vi "ActorPlugin-003-CreateWorkOrder.vi"(0 "FTW Actor Instance Configuration":string="{\n  \"Identity\": \"ActorName\",\n  \"InboxAddress\": \"tcp://127.0.0.1:*\",\n  \"PublisherAddress\": \"tcp://127.0.0.1:*\",\n  \"DebugEnableInboxLogging\": false,\n  \"DebugEnableJobLogging\": false,\n  \"DebugShowPanel\": false\n}", 11 "error in":errorcluster) -> (15 "Error":errorcluster)   [LabVIEW 2013, in "ERP-CreateWorkOrder.lvclass"]
uses:
  Actors/ERP-Create Work Order/ERP-CreateWorkOrder.lvclass
  Actors/ERP-Create Work Order/Controls/Cntrl-LoadPartNumbers.ctl
  Actors/ERP-Create Work Order/Controls/Cntrl-CreateWorkOrder.ctl
  Actors/ERP-Create Work Order/Controls/Cntrl-ClearWorkOrderVariables.ctl
  Actors/ERP-Create Work Order/ERP-CreateWorkOrder.lvclass/ERP-CreateWorkOrder.ctl
  <userlib>/_OpenG.lib/array/array.llb/Reorder 2D Array2 (String)__ogtk.vi
  ftw-dataflow/Actor/src/Instance/FTW-ActorInstance.lvclass
  ftw-dataflow/Actor/src/Message/Request/FTW-Message-IncomingRequest.lvclass
  ERP-ConfigPageNewFeather/PCert-ConfigPageNF.lvclass
panel:
  in  "Choose Part Number*":u16(ring)
  in  "Clear Work Order Variables":T1
  in  "Load Part Numbers":T2
  in  "Attach Special Instructions (Word or PDF files only!!) 2":path
  in  "Due Date*":timestamp format="%<%x>T"
  in  "Start Date*":timestamp format="%<%x>T"
  in  "Attach Special Instructions (Word or PDF files only!!) 1":path
  in  "Note - Special Instructions":string
  in  "Stage Deployment for Part":u16(ring) items=["Standard Part", "Non-Standard Part", "Inventory Part", "Waiting for Customer Supplied Material", "RMA"]
  in  "Unique Identifier":u16(ring) items=["", "Cascade", "Feinmetall", "Hermes", "Jem", "T.I.P.S"]
  in  "Type Part Number*":string
  out "Part Number Description":string
  in  "Quantity to Make*":i32
  in  "Customer*":string
  in  "Validate Typed Number":bool
  in  "Sales Order*":string
  in  "Create Work Order":T3
  # "Please Fill Out the Below Information to Create a work Order"
  # "*=Required"
  # "1."
  # "2."
  # "3."
  # "5."
  # "4."
  # "Under Construction Currently\nDoes not Work!"
  # "6."
  # "7."
  # "Drag and Drop or Select the Files to Attach"
  # "8."
  # "9."
  # "Inputs"
  # "Outputs"
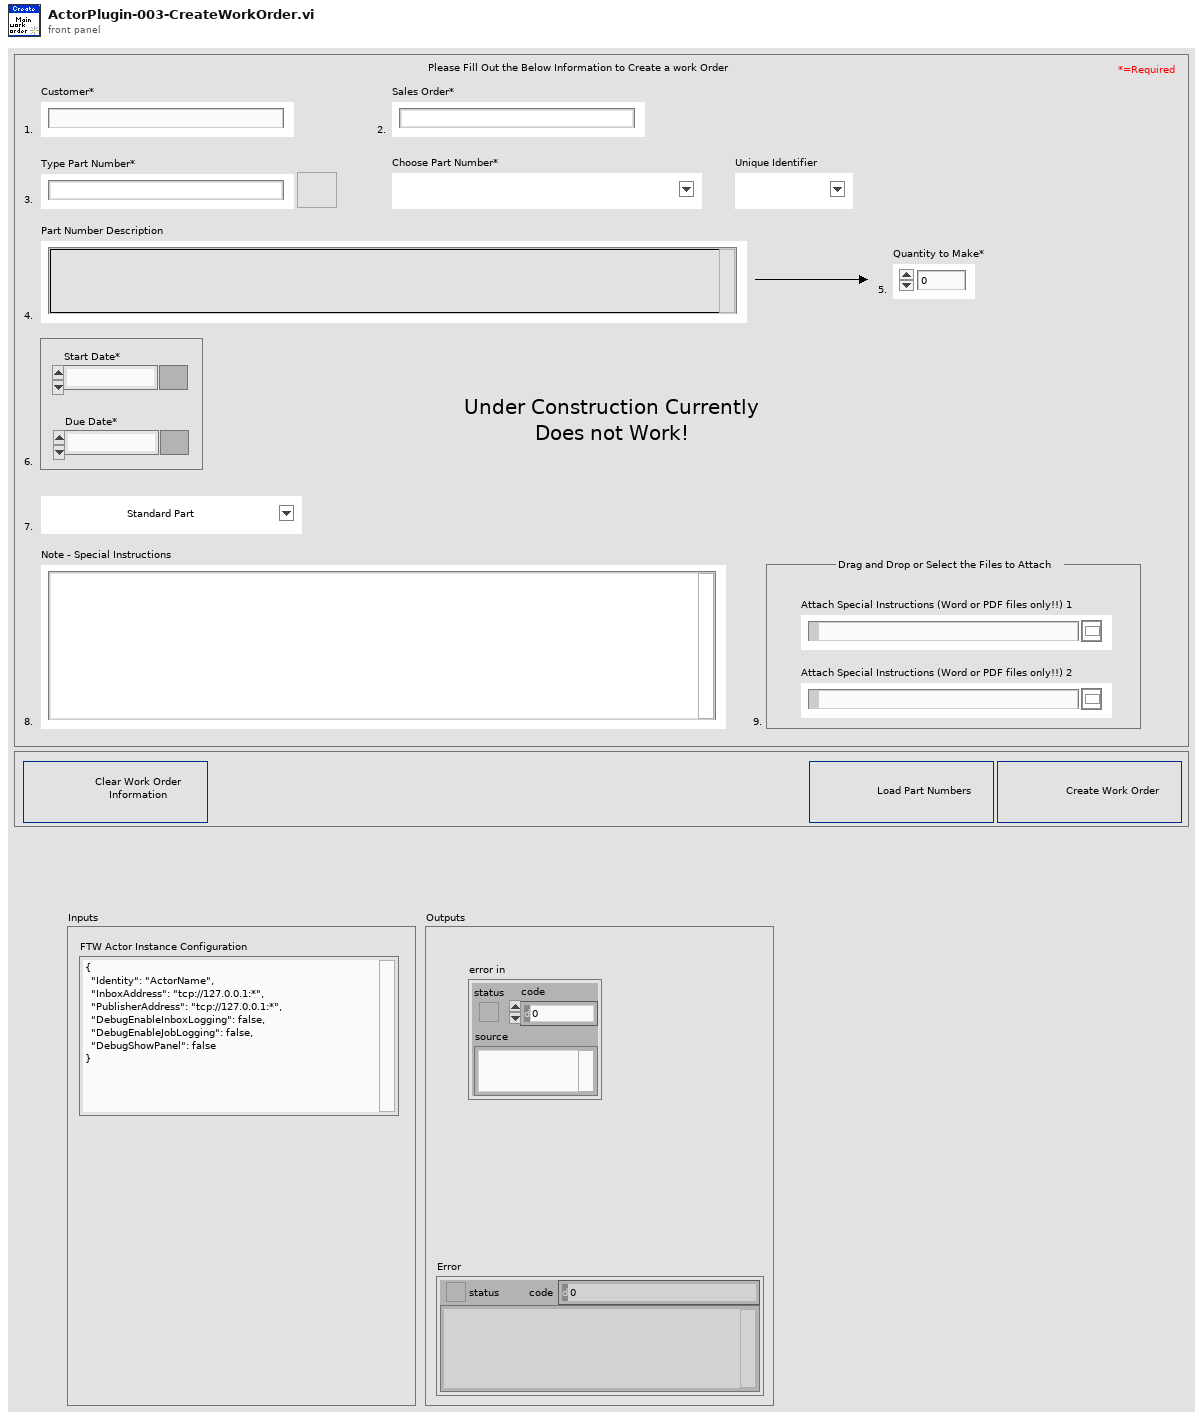
[diagram p1: front panel]
types:
  T1 = typedef "Cntrl-ClearWorkOrderVariables.ctl" = bool
  T2 = typedef "Cntrl-LoadPartNumbers.ctl" = bool
  T3 = typedef "Cntrl-CreateWorkOrder.ctl" = bool
  T4 = cluster{"Incoming Requests":refnum<event-registration>, "Additional Registration Types":refnum<event-registration>}
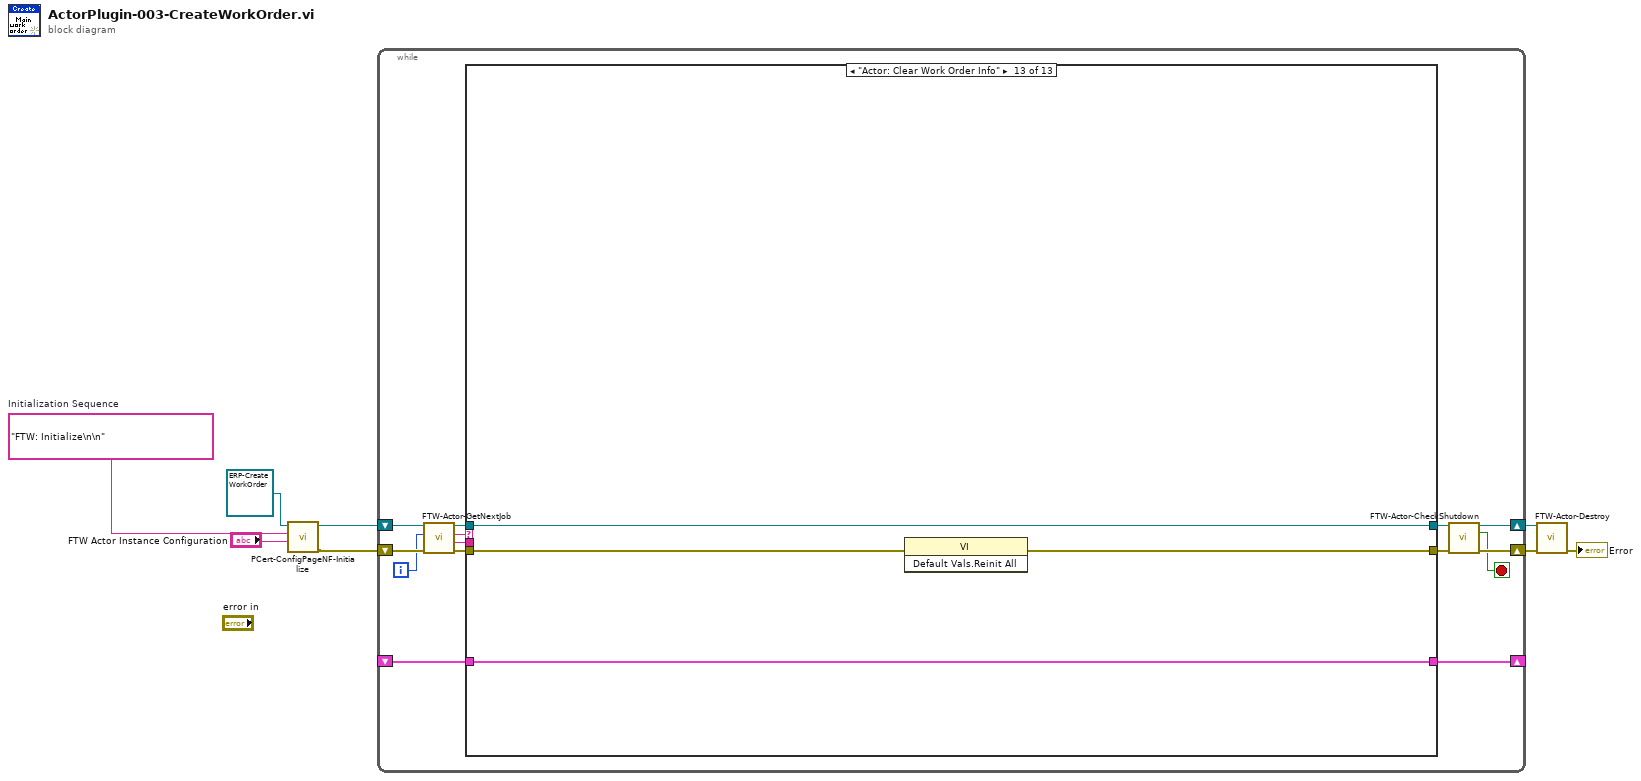
[diagram p0: block diagram]
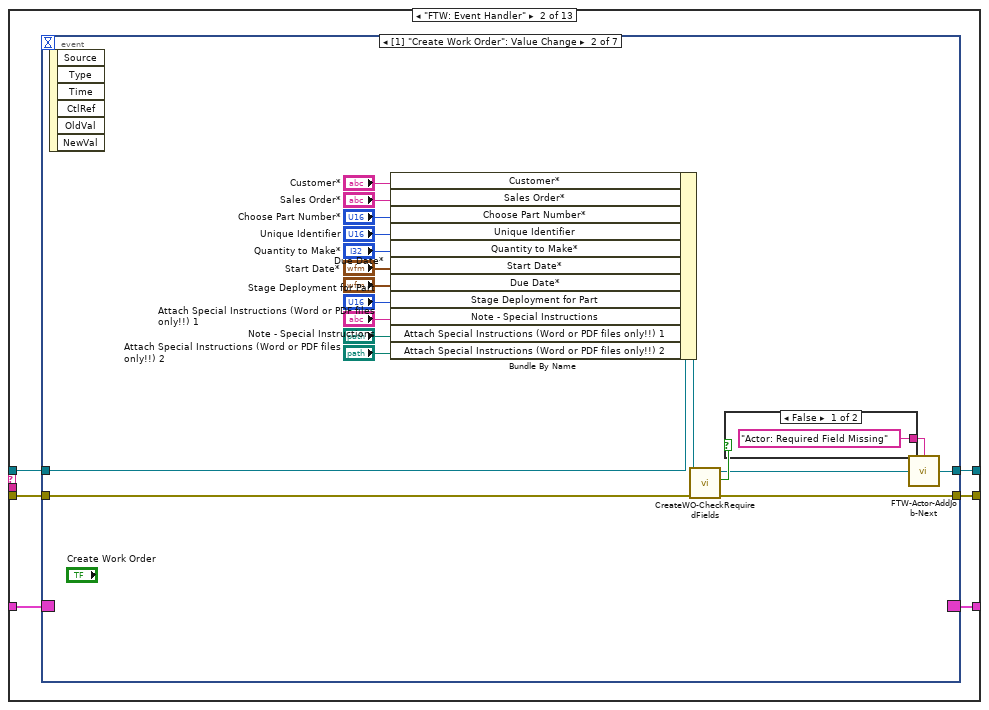
[diagram p3: hidden frame]
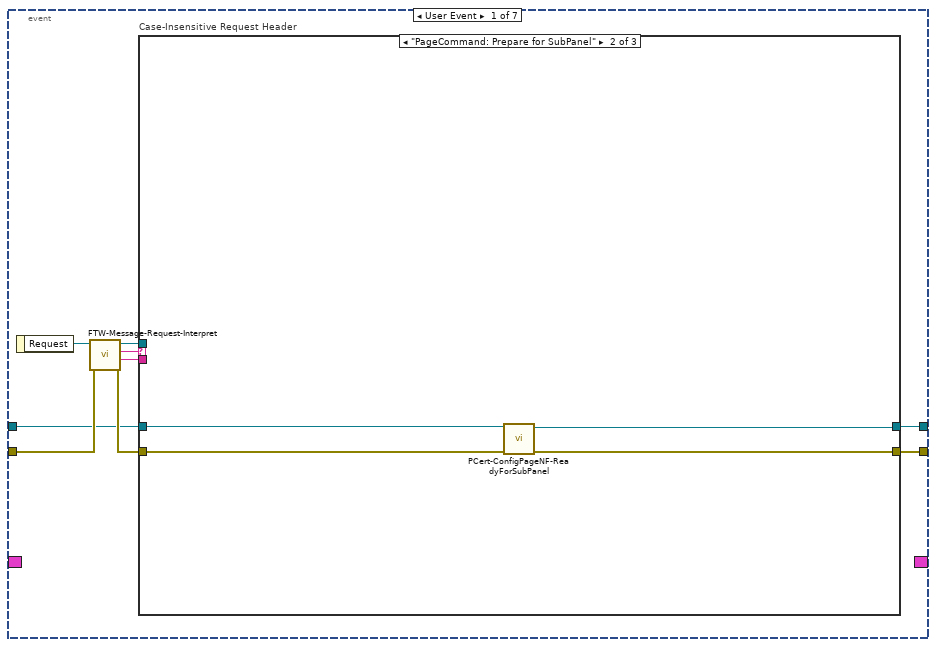
[diagram p4: hidden frame]
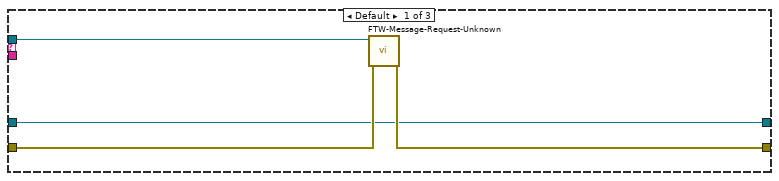
[diagram p5: hidden frame]
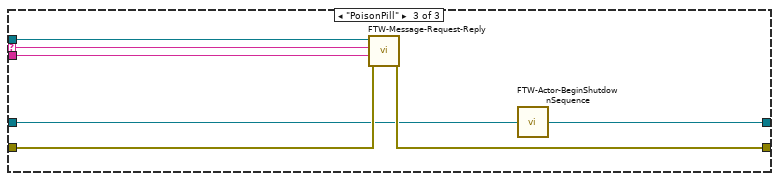
[diagram p6: hidden frame]
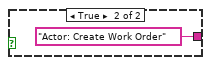
[diagram p7: hidden frame]
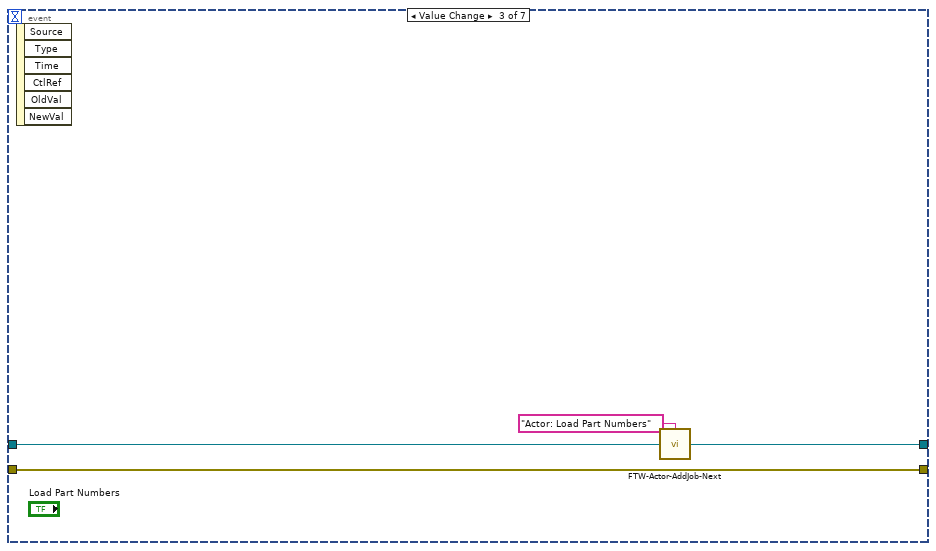
[diagram p8: hidden frame]
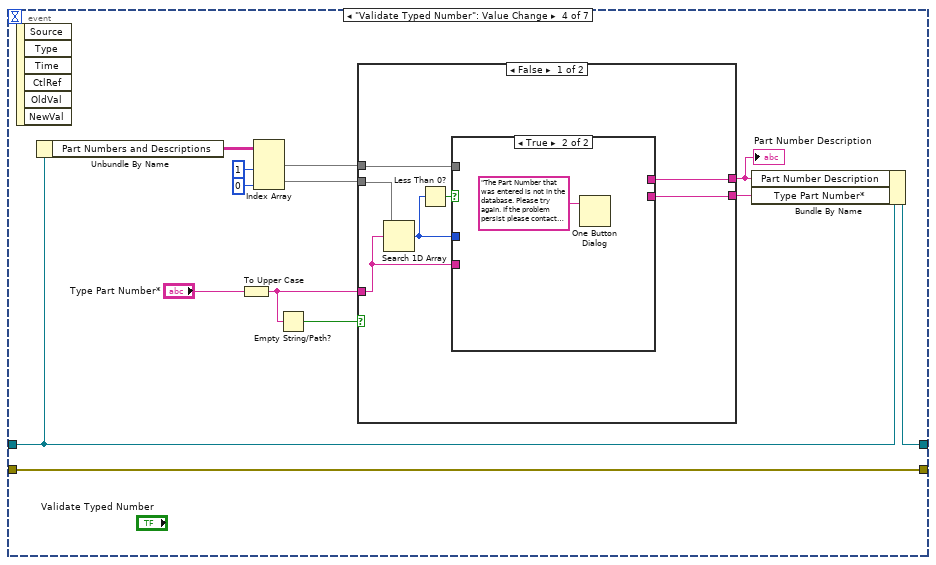
[diagram p9: hidden frame]
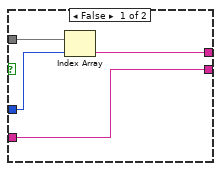
[diagram p10: hidden frame]
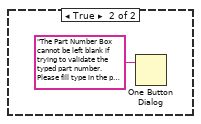
[diagram p11: hidden frame]
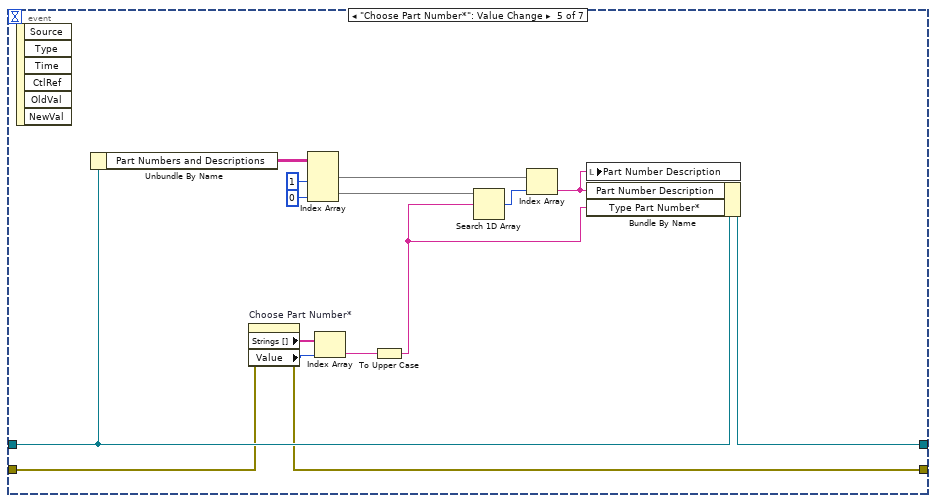
[diagram p12: hidden frame]
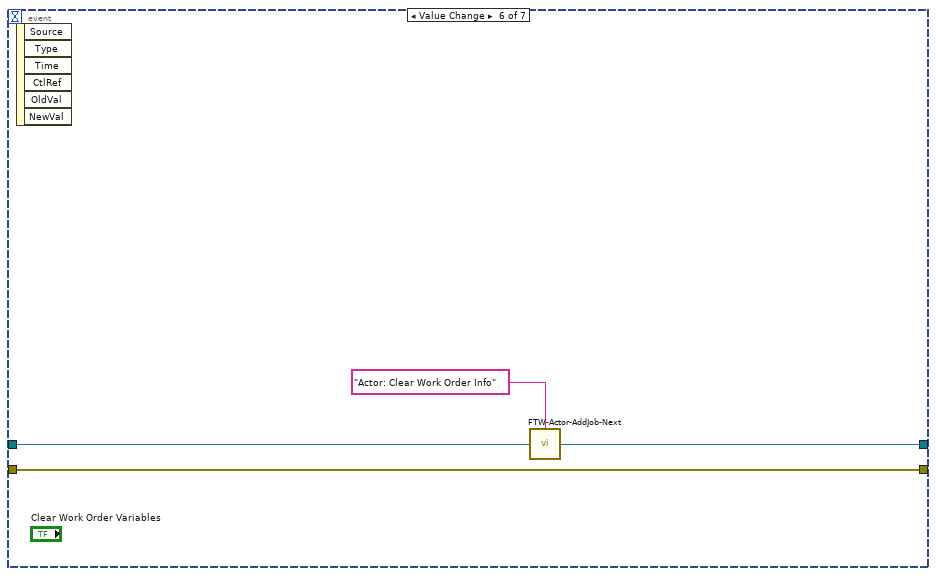
[diagram p13: hidden frame]
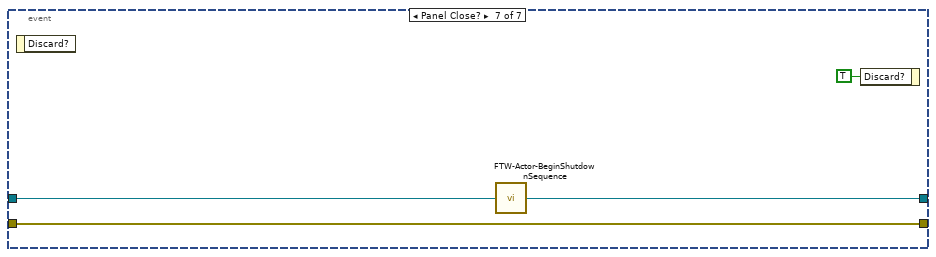
[diagram p14: hidden frame]
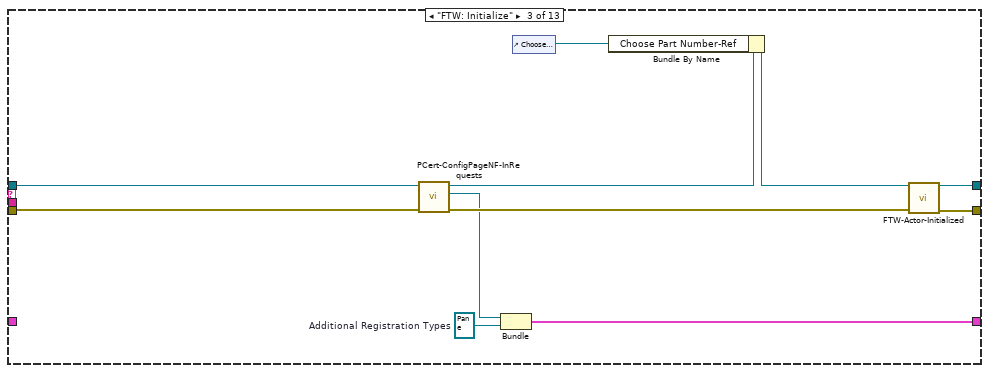
[diagram p15: hidden frame]
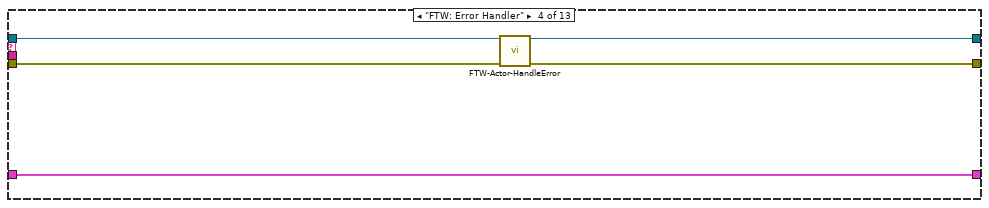
[diagram p16: hidden frame]
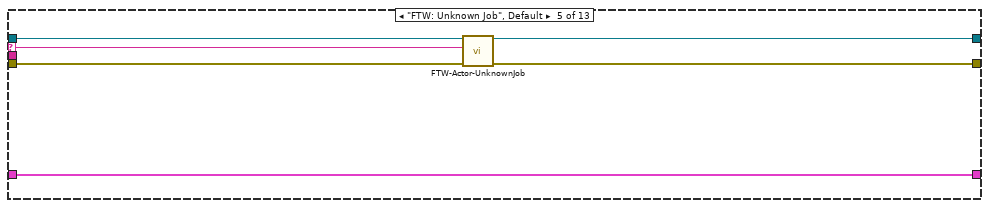
[diagram p17: hidden frame]
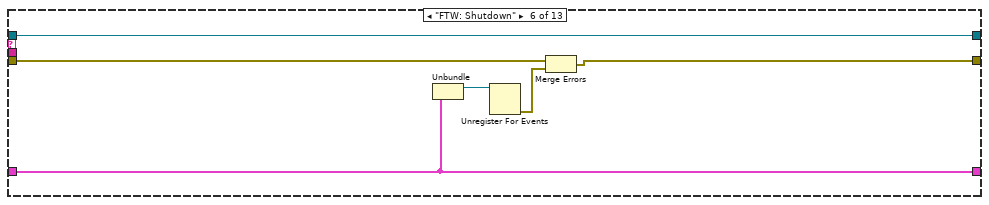
[diagram p18: hidden frame]
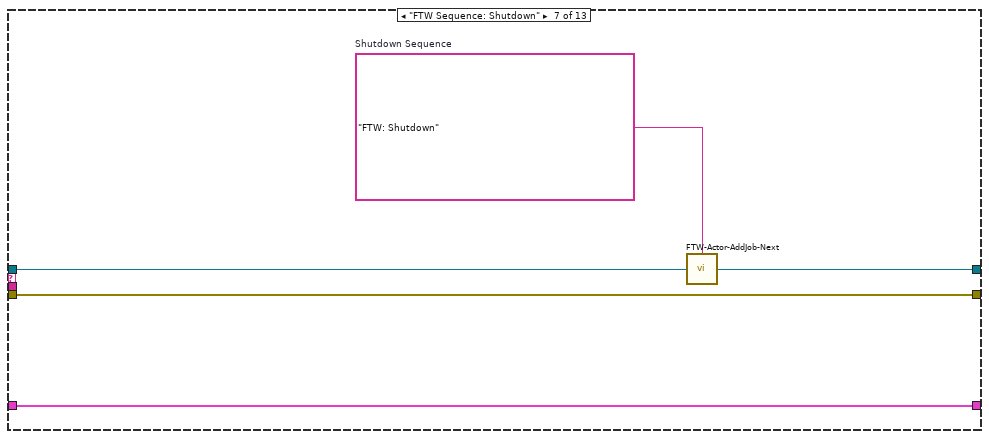
[diagram p19: hidden frame]
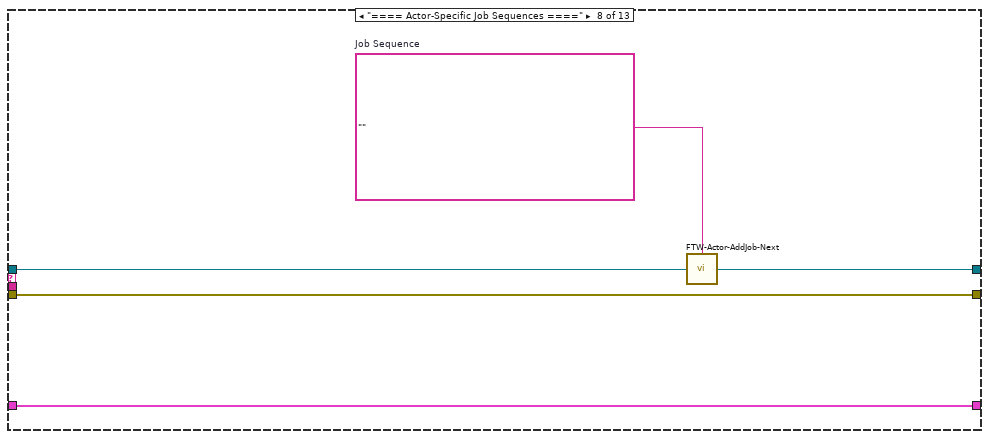
[diagram p20: hidden frame]
diagram:
  w5 = "FTW: Initialize\n\n"  # Initialization Sequence
  n1 = call-dynamic "PCert-ConfigPageNF-Initialize.vi"("FTW Actor Instance Configuration"="FTW Actor Instance Configuration", "Initialization Job Sequence"=w5, "ERP-ConfigPageNF.lvclass"=refnum<class "ERP-CreateWorkOrder.lvclass"> refnum ("ERP-CreateWorkOrder.lvclass")) -> ("error out"=w3:errorcluster, "ERP-ConfigPageNF out"=w4:refnum<class "ERP-CreateWorkOrder.lvclass">)  [unwired: 7 in]
  n2 = while {
    shift-right: [w12] -> w7
    shift-left: w3 -> [w19]
    shift-right: [w9] -> _
    shift-left: _ -> [w22]
    shift-right: [w14] -> w8
    shift-left: w4 -> [w21]
    i -> [w10]
    stop <- w11 stop-if-true
    n3 = call "FTW-Actor-GetNextJob.vi"("error in"=w19, "Jobs Performed"=w10, "FTW Actor Instance"=w21) -> ("error out"=w18:errorcluster, "Job Data"=w16:string, "Job Name"=w17:string, "FTW Actor Instance out"=w20:refnum<class "ERP-CreateWorkOrder.lvclass">)  [unwired: 5 in]
    n4 = case shown="\"Actor: Clear Work Order Info\"" w17 {
      selector: w17 -> [_ _ _ _ w146 _ _ _ _ _ _ _ _]
      tunnel: [w24 w31 w139 w141 w149 w155 w161 w166 w170 w175 w221 w224 w259] -> w13
      tunnel: w18 -> [w24 w30 w137 w143 w150 w152 w161 w166 w170 w178 w222 w233 w260]
      tunnel: w22 -> [w25 w26 _ w145 w151 w157 w162 w167 w169 w186 w223 w235 w262]
      tunnel: [w25 w29 w133 w145 w151 w157 w162 w167 w169 w186 w223 w235 w262] -> w9
      tunnel: w16 -> [_ _ _ _ _ _ _ _ _ _ _ _ _]
      tunnel: [w23 w28 w140 w142 w147 w153 w159 w164 w168 w174 w219 w225 w261] -> w15
      tunnel: w20 -> [w23 w27 w138 w144 w148 w153 w160 w165 w168 w179 w220 w234 w261]
      frame "==== Featherweight Framework Jobs ====" {
      }
      frame "FTW: Event Handler" {
        n5 = event shown="[1] \"Create Work Order\": Value Change" {
          selector: w26 -> [_ _ _ _ _ _ _]
          dyn-events: [_ _ _ _ _ _ _] -> w29
          timeout: _ -> [_ _ _ _ _ _ _]
          tunnel: [w37 w71 w80 w81 w107 w125 w128] -> w31
          tunnel: w30 -> [w38 w72 w80 w81 w109 w125 w128]
          tunnel: [w36 w58 w77 w87 w112 w122 w126] -> w28
          tunnel: w27 -> [w35 w74 w78 w88 w113 w123 w127]
          event User Event {
            n6 = event-data() -> ("Request"=w39:refnum<class "FTW-Message-IncomingRequest.lvclass">)  [unwired: 1 in]
            n7 = call "FTW-Message-Request-Interpret.vi"("error in"=w38, "FTW Incoming Request"=w39) -> ("error out"=w40:errorcluster, "Request Body"=w33:string, "Request Header"=w34:string, "FTW Incoming Request out"=w32:refnum<class "FTW-Message-IncomingRequest.lvclass">)  [unwired: 6 in]
            n8 = case "Case-Insensitive Request Header" shown="\"PageCommand: Prepare for SubPanel\"" w34 {
              selector: w34 -> [_ _ w50]
              tunnel: [w43 w47 w52] -> w37
              tunnel: w40 -> [w44 w48 w53]
              tunnel: [w41 w45 w55] -> w36
              tunnel: w35 -> [w41 w46 w51]
              tunnel: w33 -> [_ _ w49]
              tunnel: w32 -> [w42 _ w54]
              frame Default {
                n9 = call "FTW-Message-Request-Unknown.vi"("error in"=w44, "FTW Incoming Request"=w42) -> ("error out"=w43:errorcluster)  [unwired: 9 in]
              }
              frame "PageCommand: Prepare for SubPanel" {
                n10 = call "PCert-ConfigPageNF-ReadyForSubPanel.vi"("error in (no error)"=w48, "ERP-ConfigPageNF in"=w46) -> ("error out"=w47:errorcluster, "ERP-ConfigPageNF out"=w45:refnum<class "ERP-CreateWorkOrder.lvclass">)  [unwired: 8 in]
              }
              frame "PoisonPill" {
                n11 = call "FTW-Message-Request-Reply.vi"("error in"=w53, "Response Body"=w49, "Response Header"=w50, "FTW Incoming Request"=w54) -> ("error out"=w52:errorcluster)  [unwired: 6 in, 1 out]
                n12 = call "FTW-Actor-BeginShutdownSequence.vi"("FTW Actor Instance"=w51) -> ("FTW Actor Instance out"=w55:refnum<class "ERP-CreateWorkOrder.lvclass">)  [unwired: 3 in]
              }
            }
          }
          event Value Change {
            n13 = event-data() -> ()  [unwired: 1 in, 6 out]
            n14 = Bundle By Name(cluster=w74, "Customer*"="Customer*", "Sales Order*"="Sales Order*", "Choose Part Number*"="Choose Part Number*", "Unique Identifier"="Unique Identifier", "Quantity to Make*"="Quantity to Make*", "Start Date*"="Start Date*", "Due Date*"="Due Date*", "Stage Deployment for Part"="Stage Deployment for Part", "Note - Special Instructions"="Note - Special Instructions", "Attach Special Instructions (Word or PDF files only!!) 1"="Attach Special Instructions (Word or PDF files only!!) 1", "Attach Special Instructions (Word or PDF files only!!) 2"="Attach Special Instructions (Word or PDF files only!!) 2") -> (w70:refnum<class "ERP-CreateWorkOrder.lvclass">)
            n15 = call "CreateWO-CheckRequiredFields.vi"("error in (no error)"=w72, "ERP-CreateWorkOrder in"=w70) -> ("error out"=w71:errorcluster, "Create Work Order"=w60:bool, "ERP-CreateWorkOrder out"=w59:refnum<class "ERP-CreateWorkOrder.lvclass">)  [unwired: 7 in]
            n16 = case shown="False" w60 {
              tunnel: ["Actor: Required Field Missing" ("Shutdown Sequence") "Actor: Create Work Order" ("Shutdown Sequence")] -> w57
              frame False {
              }
              frame True {
              }
            }
            n17 = call "FTW-Actor-AddJob-Next.vi"("Add Next in Job Queue"=w57, "FTW Actor Instance"=w59) -> ("FTW Actor Instance out"=w58:refnum<class "ERP-CreateWorkOrder.lvclass">)  [unwired: 2 in]
          }
          event Value Change {
            n18 = event-data() -> ()  [unwired: 1 in, 6 out]
            n19 = call "FTW-Actor-AddJob-Next.vi"("Add Next in Job Queue"="Actor: Load Part Numbers" ("Shutdown Sequence"), "FTW Actor Instance"=w78) -> ("FTW Actor Instance out"=w77:refnum<class "ERP-CreateWorkOrder.lvclass">)  [unwired: 2 in]
          }
          event "Validate Typed Number": Value Change {
            n20 = event-data() -> ()  [unwired: 1 in, 6 out]
            n21 = Unbundle By Name(w88) -> ("Part Numbers and Descriptions"=w93:string[][])
            n22 = To Upper Case(1:"Type Part Number*") -> (0:w82:string)
            n23 = Index Array(array=w93, index (col) #1=1 ("disabled index (col)"), index (col) #2=0 ("index (col)")) -> (element #1=w89:string[], element #2=w90:string[])  [unwired: 2 in]
            n24 = Empty String/Path?(string/path=w82) -> (empty?=w83:bool)
            n25 = case shown="False" w83 {
              tunnel: w90 -> [w97 _]
              tunnel: w89 -> [w98 _]
              tunnel: [w95 _] -> w84
              tunnel: w82 -> [w96 _]
              tunnel: [w94 _] -> w85
              frame False {
                n26 = Search 1D Array(1D array=w97, element=w96) -> (index of element=w100:i32)  [unwired: 1 in]
                n27 = Less Than 0?(x=w100) -> (x < 0?=w99:bool)
                n28 = case shown="True" w99 {
                  tunnel: w100 -> [w103 _]
                  tunnel: w98 -> [w104 _]
                  tunnel: [w102 _] -> w95
                  tunnel: [w101 _] -> w94
                  tunnel: w96 -> [w101 _]
                  frame False {
                    n29 = Index Array(array=w104, index=w103) -> (element=w102:string)
                  }
                  frame True {
                    n30 = One Button Dialog(message="The Part Number that was entered is not in the database. Please try again. If the problem persist please contact your admin to update the database with the required part number") -> ()  [unwired: 1 in, 1 out]
                  }
                }
              }
              frame True {
                n31 = One Button Dialog(message="The Part Number Box cannot be left blank if trying to validate the typed part number. Please fill type in the part number and try again.  ") -> ()  [unwired: 1 in, 1 out]
              }
            }
            "Part Number Description" <- w84
            n32 = Bundle By Name(cluster=w88, "Part Number Description"=w84, "Type Part Number*"=w85) -> (w87:refnum<class "ERP-CreateWorkOrder.lvclass">)
          }
          event "Choose Part Number*": Value Change {
            n33 = event-data() -> ()  [unwired: 1 in, 6 out]
            n34 = Unbundle By Name(w113) -> ("Part Numbers and Descriptions"=w119:string[][])
            n35 = property on="Choose Part Number*" class="Ring (strict)"(error in=w109) -> (error out=w107:errorcluster, "Strings []"=w110:string[], "Value"=w108:u16)  [unwired: 1 in, 1 out]
            n36 = Index Array(array=w119, index (col) #1=1 ("disabled index (col)"), index (col) #2=0 ("index (col)")) -> (element #1=w116:string[], element #2=w115:string[])  [unwired: 2 in]
            n37 = Index Array(array=w110, index=w108) -> (element=w121:string)
            n38 = To Upper Case(1:w121) -> (0:w114:string)
            n39 = Search 1D Array(1D array=w115, element=w114) -> (index of element=w120:i32)  [unwired: 1 in]
            n40 = Index Array(array=w116, index=w120) -> (element=w111:string)
            n41 = local write "Part Number Description"(w111) -> ()
            n42 = Bundle By Name(cluster=w113, "Part Number Description"=w111, "Type Part Number*"=w114) -> (w112:refnum<class "ERP-CreateWorkOrder.lvclass">)
          }
          event Value Change {
            n43 = event-data() -> ()  [unwired: 1 in, 6 out]
            n44 = call "FTW-Actor-AddJob-Next.vi"("Add Next in Job Queue"="Actor: Clear Work Order Info" ("message"), "FTW Actor Instance"=w123) -> ("FTW Actor Instance out"=w122:refnum<class "ERP-CreateWorkOrder.lvclass">)  [unwired: 2 in]
          }
          event Panel Close? {
            n45 = event-data() -> ()  [unwired: 1 in, 1 out]
            n46 = call "FTW-Actor-BeginShutdownSequence.vi"("FTW Actor Instance"=w127) -> ("FTW Actor Instance out"=w126:refnum<class "ERP-CreateWorkOrder.lvclass">)  [unwired: 3 in]
            n47 = event-data("Discard?"=TRUE) -> ()  [unwired: 1 in, 1 out]
          }
        }
      }
      frame "FTW: Initialize" {
        w135 = refnum<event-registration> refnum  # Additional Registration Types
        n48 = call "PCert-ConfigPageNF-InRequests.vi"("error in (no error)"=w137, "ERP-ConfigPageNF in"=w138) -> ("error out"=w136:errorcluster, "Incoming Requests"=w134:refnum<event-registration>, "ERP-ConfigPageNF out"=w132:refnum<class "ERP-CreateWorkOrder.lvclass">)  [unwired: 7 in]
        n49 = Bundle("Incoming Requests"=w134, "Additional Registration Types"=w135) -> (w133:T4)  [unwired: 1 in]
        n50 = control-ref of="Choose Part Number*"() -> (w130:refnum<vi>)
        n51 = Bundle By Name(cluster=w132, "Choose Part Number-Ref"=w130) -> (w131:refnum<class "ERP-CreateWorkOrder.lvclass">)
        n52 = call-dynamic "FTW-Actor-Initialized.vi"("FTW Actor Instance"=w131, "error in"=w136) -> ("FTW Actor Instance out"=w140:refnum<class "ERP-CreateWorkOrder.lvclass">, "error out"=w139:errorcluster)  [unwired: 12 in]
      }
      frame "FTW: Error Handler" {
        n53 = call-dynamic "FTW-Actor-HandleError.vi"("FTW Actor Instance"=w144, "error in"=w143) -> ("FTW Actor Instance out"=w142:refnum<class "ERP-CreateWorkOrder.lvclass">, "error out"=w141:errorcluster)  [unwired: 11 in, 1 out]
      }
      frame "FTW: Unknown Job", Default {
        n54 = call-dynamic "FTW-Actor-UnknownJob.vi"("FTW Actor Instance"=w148, "Unknown Job"=w146, "error in"=w150) -> ("FTW Actor Instance out"=w147:refnum<class "ERP-CreateWorkOrder.lvclass">, "error out"=w149:errorcluster)  [unwired: 11 in]
      }
      frame "FTW: Shutdown" {
        n55 = Unbundle(w157) -> ("Incoming Requests"=w156:refnum<event-registration>)  [unwired: 1 out]
        n56 = Unregister For Events(event registration refnum=w156) -> (error out=w154:errorcluster)  [unwired: 1 in]
        n57 = Merge Errors(w152, w154) -> (w155:errorcluster)
      }
      frame "FTW Sequence: Shutdown" {
        w158 = "FTW: Shutdown"  # Shutdown Sequence
        n58 = call "FTW-Actor-AddJob-Next.vi"("Add Next in Job Queue"=w158, "FTW Actor Instance"=w160) -> ("FTW Actor Instance out"=w159:refnum<class "ERP-CreateWorkOrder.lvclass">)  [unwired: 2 in]
      }
      frame "==== Actor-Specific Job Sequences ====" {
        w163 = ""  # Job Sequence
        n59 = call "FTW-Actor-AddJob-Next.vi"("Add Next in Job Queue"=w163, "FTW Actor Instance"=w165) -> ("FTW Actor Instance out"=w164:refnum<class "ERP-CreateWorkOrder.lvclass">)  [unwired: 2 in]
      }
      frame "==== Actor-Specific Jobs ====" {
      }
      frame "Actor: Create Work Order" {
        w181 = ""
        n60 = call "JSON-ActorCommand.vi"("Payload"=w181, "error in"=w178, "Reply Command"=w181, "SQL Statement"=w181, "Table"="WorkOrders") -> ("error out"=w184:errorcluster, "Output JSON Object"=w185:string)  [unwired: 5 in]
        n61 = call "PCert-ConfigPageNF-AskDB.vi"("Timeout"=2000, "error in (no error)"=w184, "Request Body"=w185, "Request Header"="Query" ("Message Header"), "ERP-ConfigPageNF in"=w179) -> ("error out"=w177:errorcluster, "Ask Operation Failed"=w173:bool, "ERP-ConfigPageNF out"=w176:refnum<class "ERP-CreateWorkOrder.lvclass">, "Raw Data From DB"=w172:string[][])  [unwired: 2 in, 1 out]
        n62 = call "CreateWO-GenerateWorkOrder.vi"("Work Orders"=w172) -> ("Created Work Order"=w171:string)  [unwired: 8 in]
        n63 = case shown="False" w173 {
          tunnel: w177 -> [w191 w218]
          tunnel: w176 -> [w192 w217]
          tunnel: [w194 w218] -> w175
          tunnel: [w193 w217] -> w174
          tunnel: w171 -> [w190 _]
          frame False {
            n64 = call "CreateWO-WordDocumentMain.vi"("Work Order"=w190, "error in"=w191, "ERP-CreateWorkOrder in"=w192) -> ("error out"=w187:errorcluster, "Word Doc Not Created"=w189:bool, "ERP-CreateWorkOrder out"=w188:refnum<class "ERP-CreateWorkOrder.lvclass">)  [unwired: 6 in]
            n65 = case shown="False" w189 {
              tunnel: [w201 w215] -> w194
              tunnel: [w195 w214] -> w193
              tunnel: w190 -> [w208 _]
              tunnel: w188 -> [w207 w214]
              tunnel: w187 -> [w206 w215]
              frame False {
                n66 = call "CreateWO-CompileDatatoSend.vi"("Work Order"=w208, "error in"=w206, "ERP-CreateWorkOrder in"=w207) -> ("error out"=w203:errorcluster, "Output JSON to DB"=w204:string, "ERP-CreateWorkOrder out"=w205:refnum<class "ERP-CreateWorkOrder.lvclass">)  [unwired: 6 in]
                n67 = call "PCert-ConfigPageNF-AskDB.vi"("Timeout"=2000, "error in (no error)"=w203, "Request Body"=w204, "Request Header"="Insert" ("Message Header"), "ERP-ConfigPageNF in"=w205) -> ("error out"=w201:errorcluster, "ERP-ConfigPageNF out"=w196:refnum<class "ERP-CreateWorkOrder.lvclass">, "Raw Data From DB"=w199:string[][])  [unwired: 2 in, 2 out]
                n68 = Empty Array?(array=w199) -> (empty?=w198:bool)
                n69 = case shown="False" w198 {
                  tunnel: ["Actor: Clear Work Order Info" ("message") "" ("message")] -> w197
                  frame False {
                    n70 = One Button Dialog(message="Work Order Created Successfully!") -> ()  [unwired: 1 in, 1 out]
                  }
                  frame True {
                    n71 = One Button Dialog(message="Create Work Order operation has failed please try again!") -> ()  [unwired: 1 in, 1 out]
                  }
                }
                n72 = call "FTW-Actor-AddJob-Next.vi"("Add Next in Job Queue"=w197, "FTW Actor Instance"=w196) -> ("FTW Actor Instance out"=w195:refnum<class "ERP-CreateWorkOrder.lvclass">)  [unwired: 2 in]
              }
              frame True {
                n73 = One Button Dialog(message="The creation of the work order word document has failed. Please try again!") -> ()  [unwired: 1 in, 1 out]
              }
            }
          }
          frame True {
            n74 = One Button Dialog(message="Create Work Order operation has failed please try again!") -> ()  [unwired: 1 in, 1 out]
          }
        }
      }
      frame "Actor: Required Field Missing" {
        n75 = call "CreateWO-RequiredFieldsMissing.vi"("error in"=w222, "ERP-CreateWorkOrder in"=w220) -> ("error out"=w221:errorcluster, "ERP-CreateWorkOrder out"=w219:refnum<class "ERP-CreateWorkOrder.lvclass">)  [unwired: 8 in]
      }
      frame "Actor: Load Part Numbers" {
        n76 = for {
          tunnel: w234 -> [w254]
          tunnel: w233 -> [w253]
          tunnel: string[] ["ALAluminumOxideItems", "CCWItems", "ProbeCleanItems", "ProbeFormItems", "ProbeLapItems", "ProbePolishItems", "ProbeScrubItems", "OtherItems"] -> [w244] mode=indexing
          tunnel: [w251] -> w228
          shift-right: [w246] -> w226
          shift-left: string[][] [] ("reordered array") -> [w247]
          tunnel: [w245] -> w229
          shift-right: [w242] -> w227
          shift-left: string[] [] -> [w243]
          w239 = 0 ("disabled index (col)")
          w252 = ""
          n77 = call "JSON-ActorCommand.vi"("Payload"=w252, "error in"=w253, "Reply Command"=w252, "SQL Statement"=w252, "Table"=w244) -> ("error out"=w257:errorcluster, "Output JSON Object"=w258:string)  [unwired: 5 in]
          n78 = call "PCert-ConfigPageNF-AskDB.vi"("Timeout"=2000, "error in (no error)"=w257, "Request Body"=w258, "Request Header"="Query" ("Message Header"), "ERP-ConfigPageNF in"=w254) -> ("error out"=w245:errorcluster, "ERP-ConfigPageNF out"=w251:refnum<class "ERP-CreateWorkOrder.lvclass">, "Raw Data From DB"=w250:string[][])  [unwired: 2 in, 2 out]
          n79 = Build Array("" ("element"), w244) -> (w238:string[])
          n80 = call-poly <userlib>:"Reorder Array2__ogtk.vi"("reorder (rows)"=enum16{"rows", "columns"}."columns", "indices"=i32[] [0, 1], "array"=w250) -> ("reordered array"=w241:string[][])  [unwired: 8 in]
          n81 = Index Array(array=w241, index (col)=w239) -> (element=w240:string[])  [unwired: 1 in]
          n82 = Insert Into Array(array=w240, index=w239, new element=w238) -> (w237:string[])
          n83 = Insert Into Array(array=w247, new element=w241) -> (w246:string[][])  [unwired: 2 in]
          n84 = Insert Into Array(array=w243, new element=w237) -> (w242:string[])  [unwired: 1 in]
        }
        n85 = call "CreateWO-GetPartNumbers.vi"("Parts Numbers and Descriptions"=w226, "Parts Numbers"=w227, "error in (no error)"=w229, "ERP-CreateWorkOrder in"=w228) -> ("error out"=w224:errorcluster, "ERP-CreateWorkOrder out"=w225:refnum<class "ERP-CreateWorkOrder.lvclass">)  [unwired: 6 in]
      }
      frame "Actor: Clear Work Order Info" {
        n86 = invoke class="VI" method="Default Vals.Reinit All"(error in=w260) -> (error out=w259:errorcluster)  [unwired: 2 in, 2 out]
      }
    }
    n87 = call "FTW-Actor-CheckShutdown.vi"("FTW Actor Instance"=w15, "error in"=w13) -> ("FTW Actor Instance out"=w14:refnum<class "ERP-CreateWorkOrder.lvclass">, "Shutdown?"=w11:bool, "error out"=w12:errorcluster)  [unwired: 11 in]
  }
  n88 = call-dynamic "FTW-Actor-Destroy.vi"("FTW Actor Instance"=w8, "error in"=w7) -> ("error out"=→"Error":errorcluster)  [unwired: 13 in]
